vi "Scan.vi"(8 "error in":errorcluster, 10 "Scan Measurement (true)":bool=TRUE, 11 "VISA resource name":refnum<visa-resource-name>) -> (0 "error out":errorcluster, 3 "VISA resource name out":refnum<visa-resource-name>)   [LabVIEW 2017, in "Andeen-Hagerling 2700.lvlib"]
doc: "This VI Initiate or halt scan measurement."
uses:
  Andeen-Hagerling 2700.lvlib
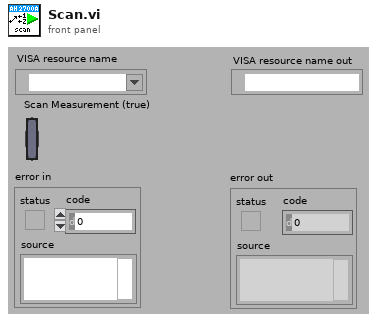
[diagram p1: front panel]
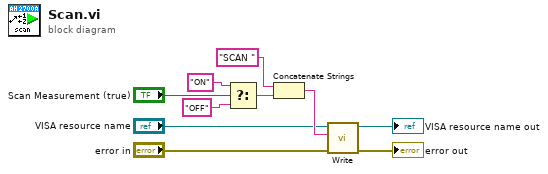
[diagram p0: block diagram]
diagram:
  n1 = Select(t="ON", s="Scan Measurement (true)", f="OFF") -> (s? t:f=w4:string)
  n2 = Concatenate Strings("SCAN " ("command"), w4) -> (w3:string)
  n3 = call "Write.vi"("error in"="error in", "command"=w3, "VISA resource name"="VISA resource name") -> ("error out"=→"error out":errorcluster, "VISA resource name out"=→"VISA resource name out":refnum<visa-resource-name>)  [unwired: 7 in]
